vi "Lex Text-Comment-Text.vi"(8 "Error In":errorcluster) -> (0 "Error Out":errorcluster)   [LabVIEW 2018, in "Tests.lvlib" / "Lexer.lvlib"]
uses:
  Lexer.lvlib
  <vilib>/addons/_JKI Toolkits/Caraya/classes/Test/Test.lvclass
  <vilib>/addons/_JKI Toolkits/Caraya/classes/Assert/Assert.lvclass
  src/Toolkit/Low-Level/Tokens/Text/Text.lvclass
  Tests.lvlib
  D:/Users/cfield/Code/Field R&D Services/Labstache/src/Toolkit/Low-Level/Tokens/Contentable/Contentable.lvclass
  D:/Users/cfield/Code/Field R&D Services/Labstache/src/Toolkit/Low-Level/Tokens/Token/Token.lvclass
  src/Toolkit/Low-Level/Support/Lex String.vi
  src/Toolkit/Low-Level/Tokens/Token/Token.lvclass
  src/Toolkit/Low-Level/Tokens/Comment/Comment.lvclass
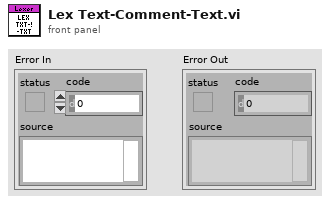
[diagram p1: front panel]
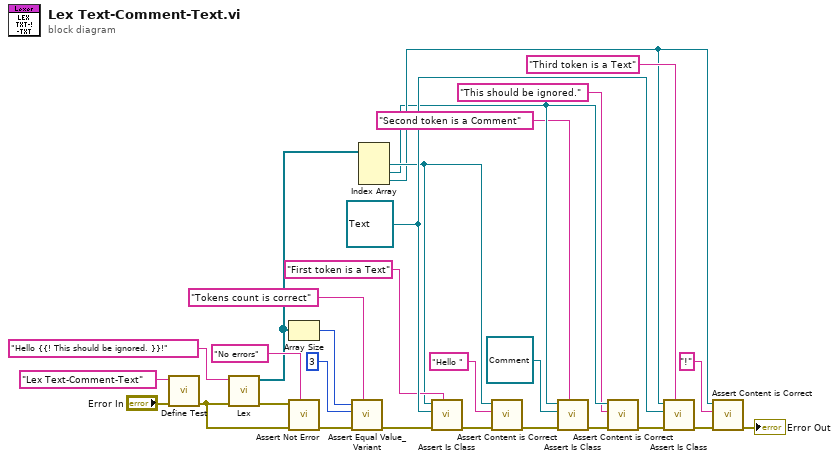
[diagram p0: block diagram]
diagram:
  w16 = refnum<class "Text.lvclass"> refnum ("Mustache.lvlib:Tokens.lvlib:Text.lvclass")
  n1 = call <vilib>:"Define Test.vi"("error in (no error)"="Error In", "Label (VI Title)"="Lex Text-Comment-Text") -> ("error out"=w9:errorcluster)  [unwired: 9 in]
  n2 = call-poly "Lex.vi"("Error In"=w9, "Input"="Hello {{! This should be ignored. }}!" ("format string")) -> ("Error Out"=w27:errorcluster, "Tokens"=w20:refnum<class "Token.lvclass">[])  [unwired: 8 in]
  n3 = Array Size(array=w20) -> (size(s)=w23:i32)
  n4 = call <vilib>:"Assert Not Error.vi"("Label"="No errors", "error in (no error)"=w9, "Not Error?"=w27) -> ("error out"=w25:errorcluster)  [unwired: 8 in]
  n5 = call <vilib>:"Assert Equal Value_Variant.vi"("Label"="Tokens count is correct", "error in (no error)"=w25, "Y"=3 ("size(s)"), "X"=w23) -> ("error out"=w21:errorcluster)  [unwired: 7 in]
  n6 = Index Array(array=w20) -> (element #1=w11:refnum<class "Token.lvclass">, element #2=w4:refnum<class "Token.lvclass">, element #3=w8:refnum<class "Token.lvclass">)  [unwired: 3 in]
  n7 = call "Assert Is Class.vi"("Label"="First token is a Text", "Error In"=w21, "Expected"=w16, "Actual"=w11) -> ("Error Out"=w19:errorcluster)  [unwired: 7 in]
  n8 = call "Assert Content is Correct.vi"("Error In"=w19, "Expected"="Hello ", "Token"=w11) -> ("Error Out"=w7:errorcluster)  [unwired: 8 in]
  n9 = call "Assert Is Class.vi"("Label"="Second token is a Comment", "Error In"=w7, "Expected"=refnum<class "Comment.lvclass"> refnum ("Toolkit.lvlib:Tokens.lvlib:Comment.lvclass"), "Actual"=w4) -> ("Error Out"=w6:errorcluster)  [unwired: 7 in]
  n10 = call "Assert Content is Correct.vi"("Error In"=w6, "Expected"="This should be ignored.", "Token"=w4) -> ("Error Out"=w5:errorcluster)  [unwired: 8 in]
  n11 = call "Assert Is Class.vi"("Label"="Third token is a Text", "Error In"=w5, "Expected"=w16, "Actual"=w8) -> ("Error Out"=w18:errorcluster)  [unwired: 7 in]
  n12 = call "Assert Content is Correct.vi"("Error In"=w18, "Expected"="!", "Token"=w8) -> ("Error Out"=→"Error Out":errorcluster)  [unwired: 8 in]
